vi "calcDemandedSteps.vi"(8 "error in (no error)":errorcluster, 9 "loopPeriod":dbl[unit]=5000.0 min=10.0 max=5000.0, 10 "step rate limit (mag)":dbl[unit]=5000000.0 min=10000.0 max=5000000.0, 11 "SystemController in":refnum<class "SystemController.lvclass">) -> (0 "error out":errorcluster, 2 "step demand":dbl=5000.0 min=10.0 max=5000.0, 3 "SystemController out":refnum<class "SystemController.lvclass">)   [LabVIEW 2013, in "SystemController.lvclass"]
uses:
  SystemController.lvclass
  SystemController.lvclass/SystemController.ctl
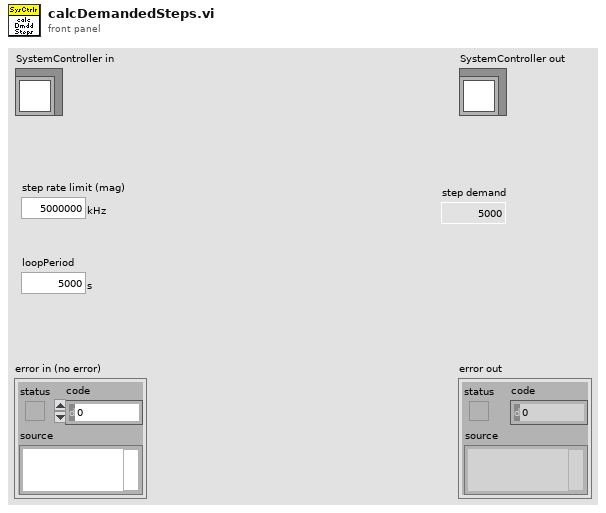
[diagram p1: front panel]
types:
  T1 = typedef "M2AADTTypedefs.lvlib/ForceDemand.ctl" = dbl[unit]
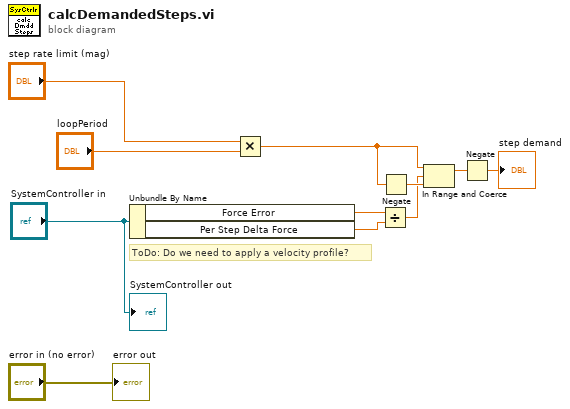
[diagram p0: block diagram]
diagram:
  # "ToDo: Do we need to apply a velocity profile?"
  n1 = Unbundle By Name("SystemController in") -> ("Force Error"=w9:T1, "Per Step Delta Force"=w8:dbl[unit])
  n2 = Multiply(x="step rate limit (mag)", y="loopPeriod") -> (x*y=w3:dbl)
  n3 = Divide(x=w9, y=w8) -> (x/y=w2:dbl)
  n4 = Negate(x=w3) -> (-x=w7:dbl)
  n5 = In Range and Coerce(upper limit=w3, x=w2, lower limit=w7) -> (coerced(x)=w6:dbl)  [unwired: 1 out]
  n6 = Negate(x=w6) -> (-x=→"step demand":dbl)
  "error out" <- "error in (no error)"
  "SystemController out" <- "SystemController in"
